vi "WPI_DashboardDelete Videos.vi"(11 "Path":path) -> ()   [LabVIEW 2025]
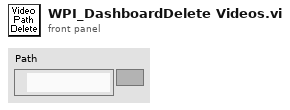
[diagram p1: front panel]
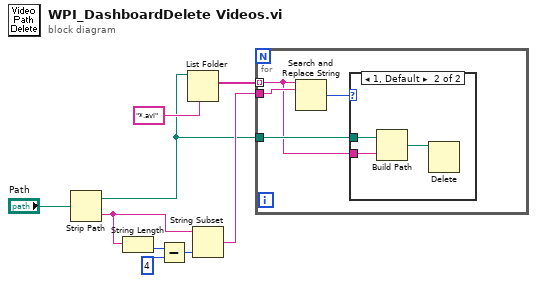
[diagram p0: block diagram]
diagram:
  n1 = Strip Path(path="Path") -> (stripped path=w2:path, name=w7:string)
  n2 = String Length(string=w7) -> (length=w8:i32)
  n3 = Subtract(x=w8, y=4) -> (x-y=w6:i32)
  n4 = List Folder(path=w2, pattern="*.avi") -> (filenames=w4:string[])  [unwired: 2 in, 3 out]
  n5 = String Subset(string=w7, length (rest)=w6) -> (substring=w5:string)  [unwired: 1 in]
  n6 = for {
    tunnel: w4 -> [w10] mode=indexing
    tunnel: w5 -> [w13]
    tunnel: w2 -> [w11]
    n7 = Search and Replace String(input string=w10, search string=w13) -> (number of replacements=w12:i32)  [unwired: 6 in, 3 out]
    n8 = case shown="1, Default" w12 {
      tunnel: w11 -> [_ w15]
      tunnel: w10 -> [_ w14]
      frame 0 {
      }
      frame 1, Default {
        n9 = Build Path(base path=w15, name or relative path=w14) -> (appended path=w16:path)
        n10 = Delete(path (use dialog)=w16) -> ()  [unwired: 4 in, 3 out]
      }
    }
  }
